vi "Secure WebSocket Server Test.vi"() -> ()   [LabVIEW 2013]
uses:
  SSL_Lib/SSL-Lib/Library Paths.ctl
  SSL Server Context/SSL Server Context.lvclass/SSL Server Context.ctl
  SSL Server Context/SSL Server Context.lvclass
  SSL Server Socket/SSL Server Socket.lvclass
  <vilib>/MediaMongrels Ltd/WebSockets/WebSockets/WebSocket Server/WebSocket Server.lvclass
  <vilib>/MediaMongrels Ltd/WebSockets/WebSockets/WebSocket/WebSocket.lvclass/WebSocket.ctl
  SSL Server Context/Write Certificate Chain File.vi
  SSL Server Context/Write Private Key.vi
  <vilib>/MediaMongrels Ltd/WebSockets/WebSockets/WebSocket/Read Return Headers.vi
  SSL_Lib/SSL-Lib/SSL-Lib.lvclass
panel:
  out "error out":errorcluster
  in  "Stop":bool
  out "Data":string
  out "Return Headers":variant
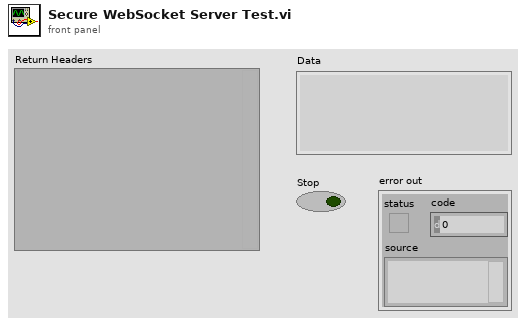
[diagram p1: front panel]
types:
  T1 = typedef "SSL_Lib.lvlib/SSL-Lib.lvclass/Library Paths.ctl" = cluster{"SSL Library Path":path, "Crypto Library Path":path}
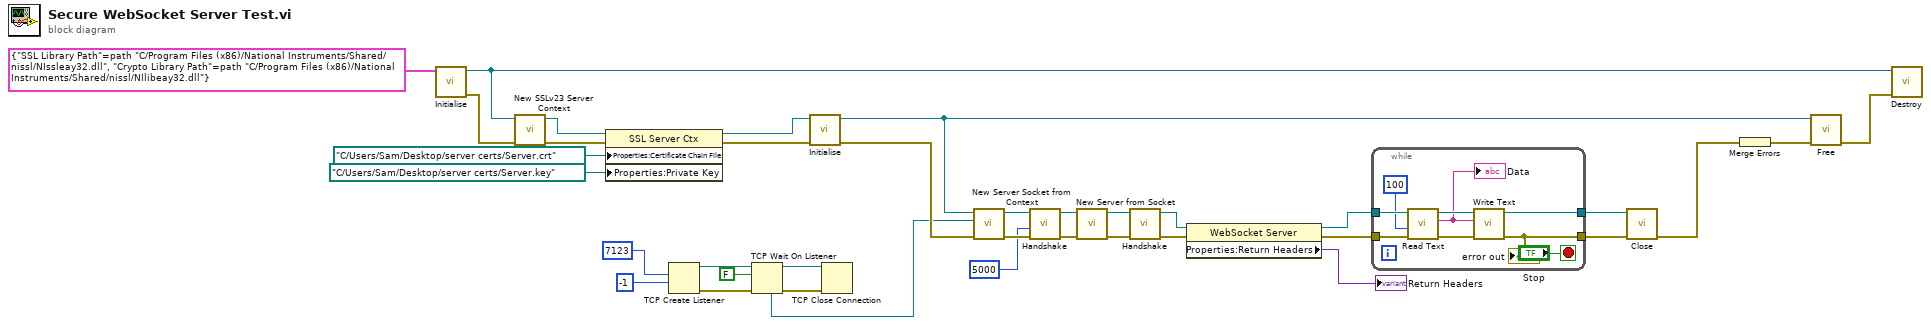
[diagram p0: block diagram]
diagram:
  n1 = call "Initialise.vi"("Library Paths"=T1 {"SSL Library Path"=path "C:/Program Files (x86)/National Instruments/Shared/nissl/NIssleay32.dll", "Crypto Library Path"=path "C:/Program Files (x86)/National Instruments/Shared/nissl/NIlibeay32.dll"}) -> ("error out"=w26:errorcluster, "SSL-Lib out"=w24:refnum<class "SSL-Lib.lvclass">)  [unwired: 9 in]
  n2 = call "New SSLv23 Server Context.vi"("error in (no error)"=w26, "SSL-Lib"=w24) -> ("error out"=w25:errorcluster, "SSL Client Context out"=w20:refnum<class "SSL Server Context.lvclass">)  [unwired: 8 in]
  n3 = property class="SSL Server Ctx"(reference=w20, error in=w25, "Properties:Certificate Chain File"=path "C:/Users/Sam/Desktop/server certs/Server.crt", "Properties:Private Key"=path "C:/Users/Sam/Desktop/server certs/Server.key") -> (reference out=w19:refnum<class "SSL Server Context.lvclass">, error out=w21:errorcluster)
  n4 = TCP Create Listener(9:-1 ("timeout ms (25000)"), 10:u16 7123 ("port")) -> (0:w7:errorcluster, 3:w10:refnum<k5>)  [unwired: 3 in, 1 out]
  n5 = TCP Wait On Listener(8:w7, 10:FALSE ("resolve remote address (T)"), 11:w10) -> (0:w9:errorcluster, 3:w8:refnum<k5>, 4:w1:refnum<k5>)  [unwired: 1 in, 2 out]
  n6 = call-dynamic "Initialise.vi"("error in (no error)"=w21, "OpenSSL Server Context in"=w19) -> ("error out"=w17:errorcluster, "OpenSSL Server Context out"=w18:refnum<class "SSL Server Context.lvclass">)  [unwired: 8 in]
  n7 = TCP Close Connection(connection ID=w8, error in (no error)=w9) -> ()  [unwired: 1 in, 2 out]
  n8 = call "New Server Socket from Context.vi"("error in (no error)"=w17, "TCP Refnum"=w1, "SSL Server Ctx"=w18) -> ("error out"=w5:errorcluster, "SSL Server Skt out"=w6:refnum<class "SSL Server Socket.lvclass">)  [unwired: 7 in]
  n9 = call-dynamic "Handshake.vi"("error in (no error)"=w5, "Timeout (5000ms)"=u32 5000, "OpenSSL in"=w6) -> ("error out"=w4:errorcluster, "OpenSSL out"=w3:refnum<class "SSL Server Socket.lvclass">)  [unwired: 7 in]
  n10 = call <vilib>:"New Server from Socket.vi"("error in (no error)"=w4, "Socket"=w3) -> ("error out"=w36:errorcluster, "WebSocket Server out"=w35:refnum<class "WebSocket Server.lvclass">)  [unwired: 8 in]
  n11 = call-dynamic "Handshake.vi"("error in (no error)"=w36, "WebSocket Connection in"=w35) -> ("error out"=w34:errorcluster, "WebSocket Connection out"=w33:refnum<class "WebSocket Server.lvclass">)  [unwired: 8 in]
  n12 = property class="WebSocket Server"(reference=w33, error in=w34) -> (reference out=w30:refnum<class "WebSocket Server.lvclass">, error out=w31:errorcluster, "Properties:Return Headers"=→"Return Headers":variant)
  n13 = while {
    tunnel: w31 -> [w45]
    tunnel: w30 -> [w44]
    tunnel: [w41] -> w29
    tunnel: [w40] -> w28
    stop <- "Stop" stop-if-true
    n14 = call-dynamic "Read Text.vi"("error in (no error)"=w45, "timeout ms (5000)"=100, "WebSocket in"=w44) -> ("error out"=w43:errorcluster, "Data"=w39:string, "WebSocket out"=w42:refnum<class "WebSocket Server.lvclass">)  [unwired: 6 in]
    "Data" <- w39
    n15 = call-dynamic "Write Text.vi"("error in (no error)"=w43, "String Data"=w39, "WebSocket in"=w42) -> ("error out"=w41:errorcluster, "WebSocket out"=w40:refnum<class "WebSocket Server.lvclass">)  [unwired: 7 in]
    "error out" <- w41
  }
  n16 = call-dynamic "Close.vi"("error in (no error)"=w29, "WebSocket in"=w28) -> ("error out"=w22:errorcluster)  [unwired: 9 in]
  n17 = Merge Errors(w22) -> (w16:errorcluster)
  n18 = call-dynamic "Free.vi"("error in (no error)"=w16, "OpenSSL Context in"=w18) -> ("error out"=w23:errorcluster)  [unwired: 9 in]
  n19 = call "Destroy.vi"("error in (no error)"=w23, "SSL-Lib in"=w24) -> ()  [unwired: 9 in, 1 out]
